vi "IP to String 2.vi"(11 "Start IP":u8[](array[numeric])=[169, 254, 146, 100]) -> (3 "resulting string":string)   [LabVIEW 2022 SP3]
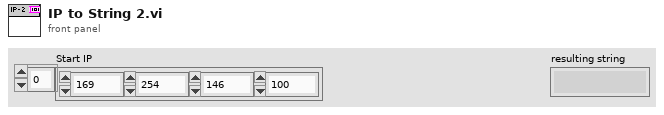
[diagram p1: front panel]
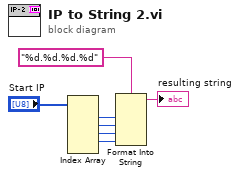
[diagram p0: block diagram]
diagram:
  n1 = Index Array(array="Start IP") -> (element #1=w5:u8, element #2=w4:u8, element #3=w3:u8, element #4=w2:u8)  [unwired: 5 in, 1 out]
  n2 = Format Into String(format string="%d.%d.%d.%d", w5, w4, w3, w2) -> (resulting string=→"resulting string":string)  [unwired: 2 in, 1 out]
